vi "Actor Core.vi"(8 "error in":errorcluster, 11 "RP I-V in":refnum<class "RP I-V.lvclass">) -> (0 "error out":errorcluster, 3 "Actor out":refnum<class "Actor.lvclass">)   [LabVIEW 2016, in "RP I-V.lvclass"]
doc: "(<B>Filename</B>: Actor Framework.lvlib:Actor.lvclass:Actor Core.vi)\n\nReceives messages to the actor, reacts to them, and initiates any error handling that may shut the actor down.\n\nDescendant classes may override this VI to append parallel tasks for the actor to complete while it handles messages. Overrides use the Call Parent Method node."
uses:
  RP I-V.lvclass
  <vilib>/ActorFramework/Actor/Actor.lvclass
  NHMFL_Core/Libraries/Red Pitaya/RP Core/Rep Pitaya I-V driver/RP I-V Configuration.ctl
  NHMFL_Core/Libraries/Instruments/Pulse Driver/Pusle Driver Configuration.ctl
  NHMFL_Core/Libraries/Red Pitaya/Waform generation/I-V parameters.ctl
  Measure_core/Pulse Recorders/Pulse Recorder/Pulse Recorder.lvclass
panel:
  out "Armed":bool
  out "Name":string
  in  "Configuration":T1={"Recorder"={"Pre-trigger duration"=0.01, "Post-trigger duration"=0.1, "Rate"=1000000.0, "Ranges"=[10.0], "Re-name channels"=[], "Active channels"="0:1", "External clock"=FALSE}, "I-V parameters"={"Start magnitude"=2e-05, "Magnitude increment"=5e-05, "Number of pulses"=50, "Baseline length"=0, "Ramp length"=0, "Top  length"=0, "Threshold "=2e-06, "Processing Delay"=255, "Valhalla range"=0.001, "Interpolation"=64}} {"Recorder"."Rate" format="%#_8pHz"; "Recorder"."Post-trigger duration" format="%#_6ps"; "Recorder"."Pre-trigger duration" format="%#_6ps"; "Recorder"."Ranges" format="%#_6pV"; "I-V parameters"."Valhalla range" format="%#_6pA"; "I-V parameters"."Processing Delay" format="%dpts"; "I-V parameters"."Threshold" format="%#_6pV"; "I-V parameters"."Top  length" format="%dpts"; "I-V parameters"."Ramp length" format="%dpts"; "I-V parameters"."Baseline length" format="%dpts"; "I-V parameters"."Magnitude increment" format="%#_6pA"; "I-V parameters"."Start magnitude" format="%#_6pA"}
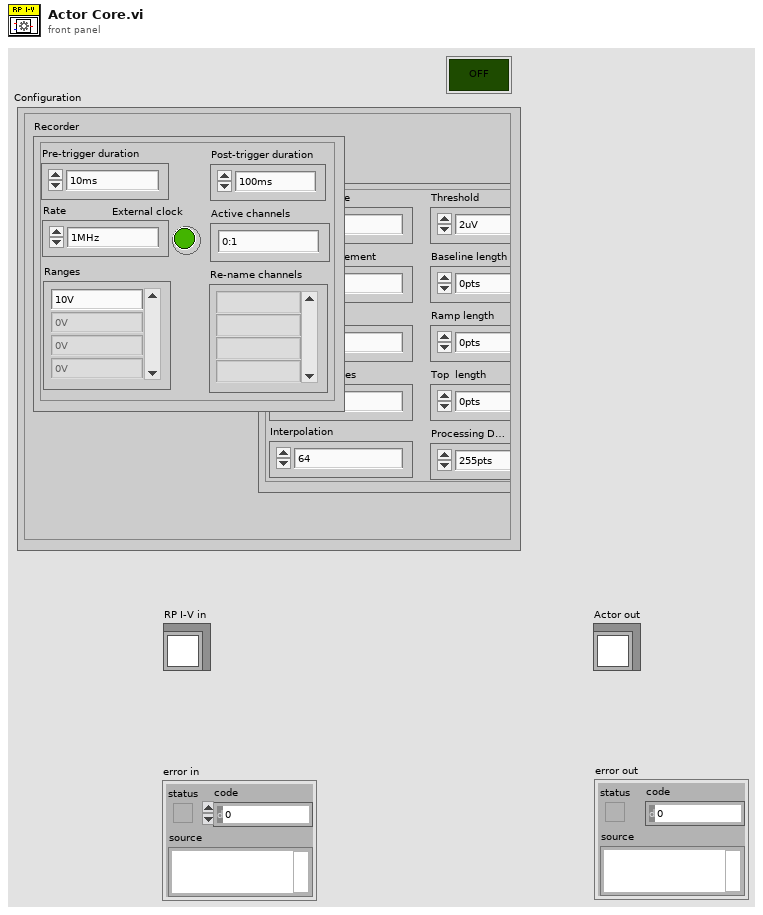
[diagram p1: front panel]
types:
  T1 = typedef "RP I-V Configuration.ctl" = cluster{"Recorder":T2, "I-V parameters":T3}
  T2 = typedef "Pusle Driver Configuration.ctl" = cluster{"Pre-trigger duration":dbl, "Post-trigger duration":dbl, "Rate":dbl, "Ranges":dbl[], "Re-name channels":string[], "Active channels":string, "External clock":bool}
  T3 = typedef "I-V parameters.ctl" = cluster{"Start magnitude":dbl, "Magnitude increment":dbl, "Number of pulses":i32, "Baseline length":i32, "Ramp length":i32, "Top  length":i32, "Threshold ":dbl, "Processing Delay":u16, "Valhalla range":dbl, "Interpolation":i32}
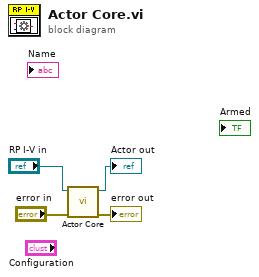
[diagram p0: block diagram]
diagram:
  n1 = call-parent "Actor Core.vi"("error in"="error in", "Pulse Recorder in"="RP I-V in") -> ("error out"=→"error out":errorcluster, "Actor out"=→"Actor out":refnum<class "Actor.lvclass">)  [unwired: 8 in]
